vi "Measure Targets.vi"(11 "Unmeasured Targets in":T1[](array[typedef])) -> (3 "Measured Targets out":T1[](array[typedef]))   [LabVIEW 2014]
uses:
  Vision Tote Data.ctl
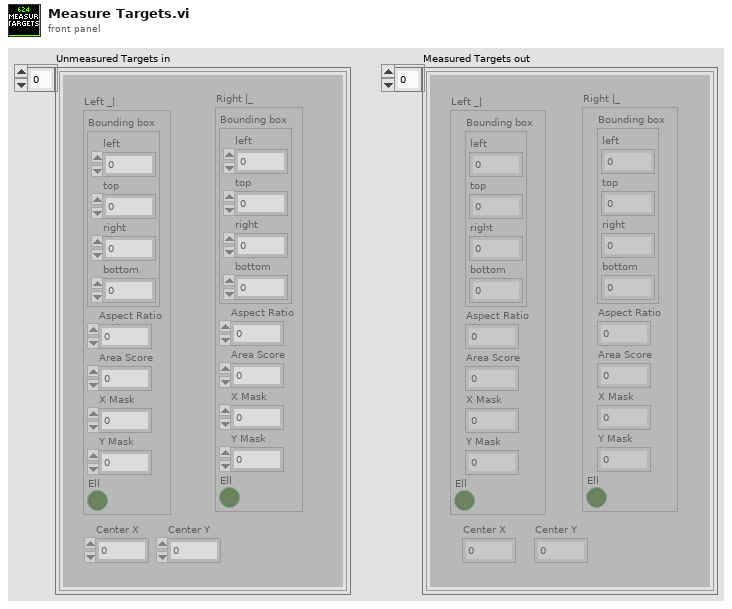
[diagram p1: front panel]
types:
  T1 = typedef "Vision Tote Data.ctl" = cluster{"Left _|":cluster{"Bounding box":cluster{"left":dbl, "top":dbl, "right":dbl, "bottom":dbl}, "Aspect Ratio":dbl, "Area Score":dbl, "X Mask":dbl, "Y Mask":dbl, "Ell":bool}, "Right |_":cluster{"Bounding box":cluster{"left":dbl, "top":dbl, "right":dbl, "bottom":dbl}, "Aspect Ratio":dbl, "Area Score":dbl, "X Mask":dbl, "Y Mask":dbl, "Ell":bool}, "Center X":dbl, "Center Y":dbl}
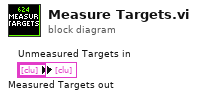
[diagram p0: block diagram]
diagram:
  "Measured Targets out" <- "Unmeasured Targets in"
